vi "Add Section.vi"(8 "error in":errorcluster, 10 "Section Node":refnum<k20>, 11 "Item Ref in":refnum<data-value>) -> (0 "error out":errorcluster, 3 "Item Ref out":refnum<data-value>)   [LabVIEW 2024, in "Config File Parser.lvlib" / "Section.lvclass"]
uses:
  Section.lvclass
  Item/Item.lvclass
  Item/Item Type.ctl
  Config File Parser.lvlib
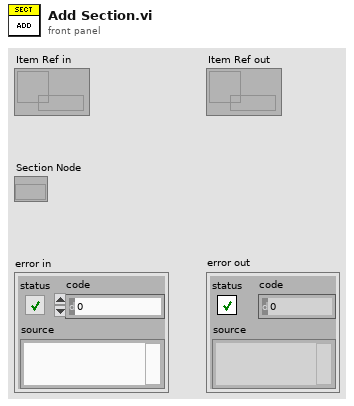
[diagram p1: front panel]
types:
  T1 = typedef "Config File Parser.lvlib/Item.lvclass/Item Type.ctl" = enum16{"Property", "Channel", "Section"}
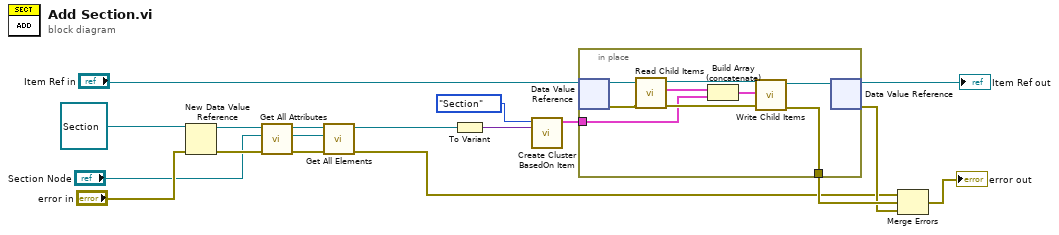
[diagram p0: block diagram]
diagram:
  n1 = New Data Value Reference(data value=refnum<class "Section.lvclass"> refnum ("Section.lvclass"), error in="error in") -> (data value reference=w1:refnum<data-value>, error out=w13:errorcluster)
  n2 = call "Get All Attributes.vi"("error in"=w13, "Section Node"="Section Node", "Section Ref in"=w1) -> ("error out"=w12:errorcluster, "Section Ref out"=w4:refnum<data-value>)  [unwired: 7 in]
  n3 = call "Get All Elements.vi"("error in"=w12, "Section Node"="Section Node", "Section Ref in"=w4) -> ("error out"=w11:errorcluster, "Section Ref out"=w3:refnum<data-value>)  [unwired: 7 in]
  n4 = To Variant(anything=w3) -> (Variant=w6:variant)
  n5 = call "Create Cluster BasedOn Item.vi"("Item Value"=w6, "Item Type"=Item_Type."Section" ("Type")) -> ("Cluster"=w10:cluster{"Type":T1, "Value":variant})  [unwired: 9 in]
  n6 = in-place {
    in-place-border: w10 -> [w20]
    in-place-border: [w24] -> w16
    n7 = in-place-dvr #1("Item Ref in") -> (w19:refnum<class "Item.lvclass">, w25:errorcluster)
    n8 = call-dynamic "Read Child Items.vi"("error in"=w25, "Item in"=w19) -> ("error out"=w26:errorcluster, "Child Items"=w23:cluster{"Type":T1, "Value":variant}[], "Item out"=w21:refnum<class "Item.lvclass">)  [unwired: 7 in]
    n9 = Build Array (concatenate)(w23, w20) -> (w22:cluster{"Type":T1, "Value":variant}[])
    n10 = call-dynamic "Write Child Items.vi"("error in"=w26, "Child Items"=w22, "Item in"=w21) -> ("error out"=w24:errorcluster, "Item out"=w18:refnum<class "Item.lvclass">)  [unwired: 7 in]
    n11 = in-place-dvr #1(w18) -> (→"Item Ref out":refnum<data-value>, w15:errorcluster)
  }
  n12 = Merge Errors(w11, w16, w15) -> (→"error out":errorcluster)
